vi "Read S_0.vi"(8 "error in (no error)":errorcluster, 11 "Analytical Serial Arm Class in":refnum<class "NI_Robotics_Analytical Serial Arm Class.lvclass">) -> (0 "error out":errorcluster, 2 "S_0":dbl, 3 "Analytical Serial Arm Class out":refnum<class "NI_Robotics_Analytical Serial Arm Class.lvclass">)   [LabVIEW 2017, in "NI_Robotics_Analytical Serial Arm Class.lvclass"]
uses:
  <vilib>/robotics/Kinematics/Analytical/Generic/NI_Robotics_Analytical Serial Arm Class.lvclass
  <vilib>/robotics/Kinematics/Analytical/Generic/NI_Robotics_Analytical Serial Arm Class.lvclass/NI_Robotics_Analytical Serial Arm Class.ctl
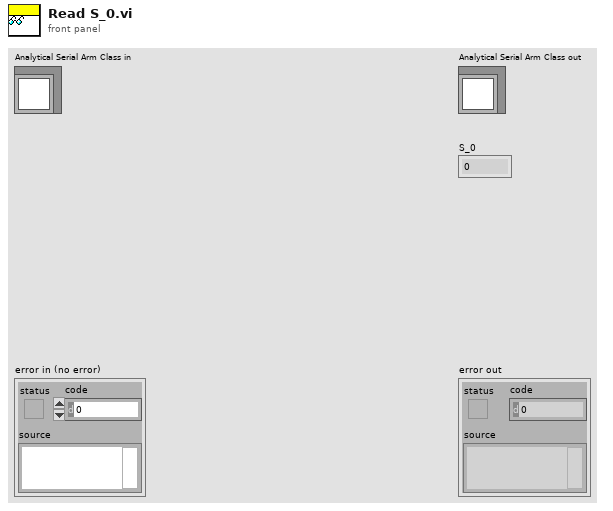
[diagram p1: front panel]
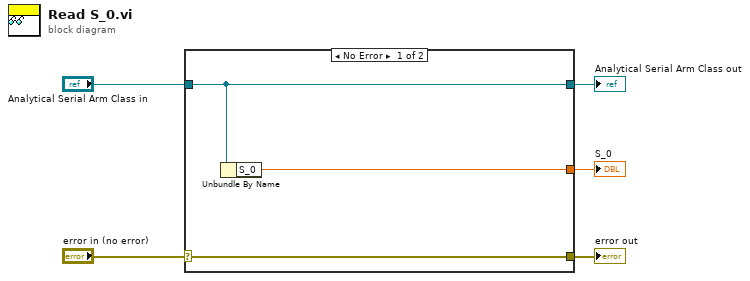
[diagram p0: block diagram]
diagram:
  n1 = case shown="No Error" "error in (no error)" {
    selector: "error in (no error)" -> [w8 w9]
    tunnel: [w8 w9] -> w4
    tunnel: [w7 w10] -> w2
    tunnel: "Analytical Serial Arm Class in" -> [w7 w10]
    tunnel: [w6 _] -> w1
    frame No Error {
      n2 = Unbundle By Name(w7) -> ("S_0"=w6:dbl)
    }
    frame Error {
    }
  }
  "error out" <- w4
  "Analytical Serial Arm Class out" <- w2
  "S_0" <- w1
